vi "Global Variables.vi"() -> ()   [LabVIEW 2018]
panel:
  out "TabletProtocol":string
  out "FanProtocol":string
  out "ResistanceProtocol":string
  out "GradeProtocol":string
  out "DistanceDriver":string
  out "SpeedProtocol":string
  out "EnabledUSB":string
  in  "xmlParser 3":string[](array[string])=["Enabled", "SpeedProtocol", "DistanceDriver", "GradeProtocol", "ResistanceDriver", "FanProtocol", "TabletProtocol"]
  out "TVTest":string
  out "USBTest":string
  out "SoftwareVersion":string
  out "InclineCalibration":string
  out "Cosmetic":string
  out "Warning":string
  out "Finish":string
  out "CSAFETest":string
  out "AudioTest":string
  out "FanTest":string
  out "PulseTest":string
  out "ResistanceTest":string
  out "InclineTest":string
  out "TachInputTest":string
  out "PWMTest":string
  out "ButtonTest":string
  out "DisplayTest":string
  out "SafetyKey":string
  out "PowerUp":string
  out "Setup":string
  out "EquipmentNeeded":string
  out "BLETest":string
  out "BLESetup":string
  out "Firmware":string
  out "DisplayType":string
  out "CurrentLimit":string
  out "ConsoleVoltage":string
  out "Controller":string
  out "Description":string
  out "Units":string
  out "ProductType":string
  out "MCU":string
  out "PartNumber":string
  out "xPulse":i32
  out "yTV":i32
  out "xTV":i32
  out "yAudio":i32
  out "xAudio":i32
  out "y2Pulse":i32
  out "y1Pulse":i32
  out "advanceButton":i32
  out "modeButton":i32
  out "xmlFeature2":string[][](array[string])
  out "xmlData":string[](array[string])
  out "xmlFeature1":string[](array[string])
  in  "xmlParser 2":string[](array[string])=["MaxSpeed", "MinGrade", "MaxGrade", "TransMax", "DistanceDriver", "FanProtocol", "TabletProtocol"]
  in  "xmlParser 1":string[](array[string])=["consolePartNumber", "mcuChipName", "equipmentType", "systemUnitType", "BuildModelString", "PowerBoard", "ConsoleVoltage", "MaxCurrent"]
  in  "xmlParser 0":string[](array[string])=["SystemInfo/", "Display/TypeName", "ReleaseArray/ReleaseItem/GithubLink", "FeatureArray/FeatureItem", "FeatureArray/FeatureItem/", "KeyArray/KeyObj/MembraneKeyCode/KeyCodeValue", "AudioSources/AudioSrcItem", "PulseDriverArray/PulseDriverItem"]
  in  "jsonGen":string[](array[string])=["PartNumber", "Description", "ProductType", "DisplayType", "EquipmentNeeded", "Setup", "BLESetup", "Cosmetic", "PowerUp", "SafetyKey", "BLETest", "SoftwareVersion", "InclineCalibration", "DisplayTest", "ButtonTest", "PWMTest", "TachInputTest", "InclineTest", "ResistanceTest", "USBTest", "PulseTest", "FanTest", "AudioTest", "TVTest", "CSAFETest", "Finish"]
  # "Not used. Save this for other functions"
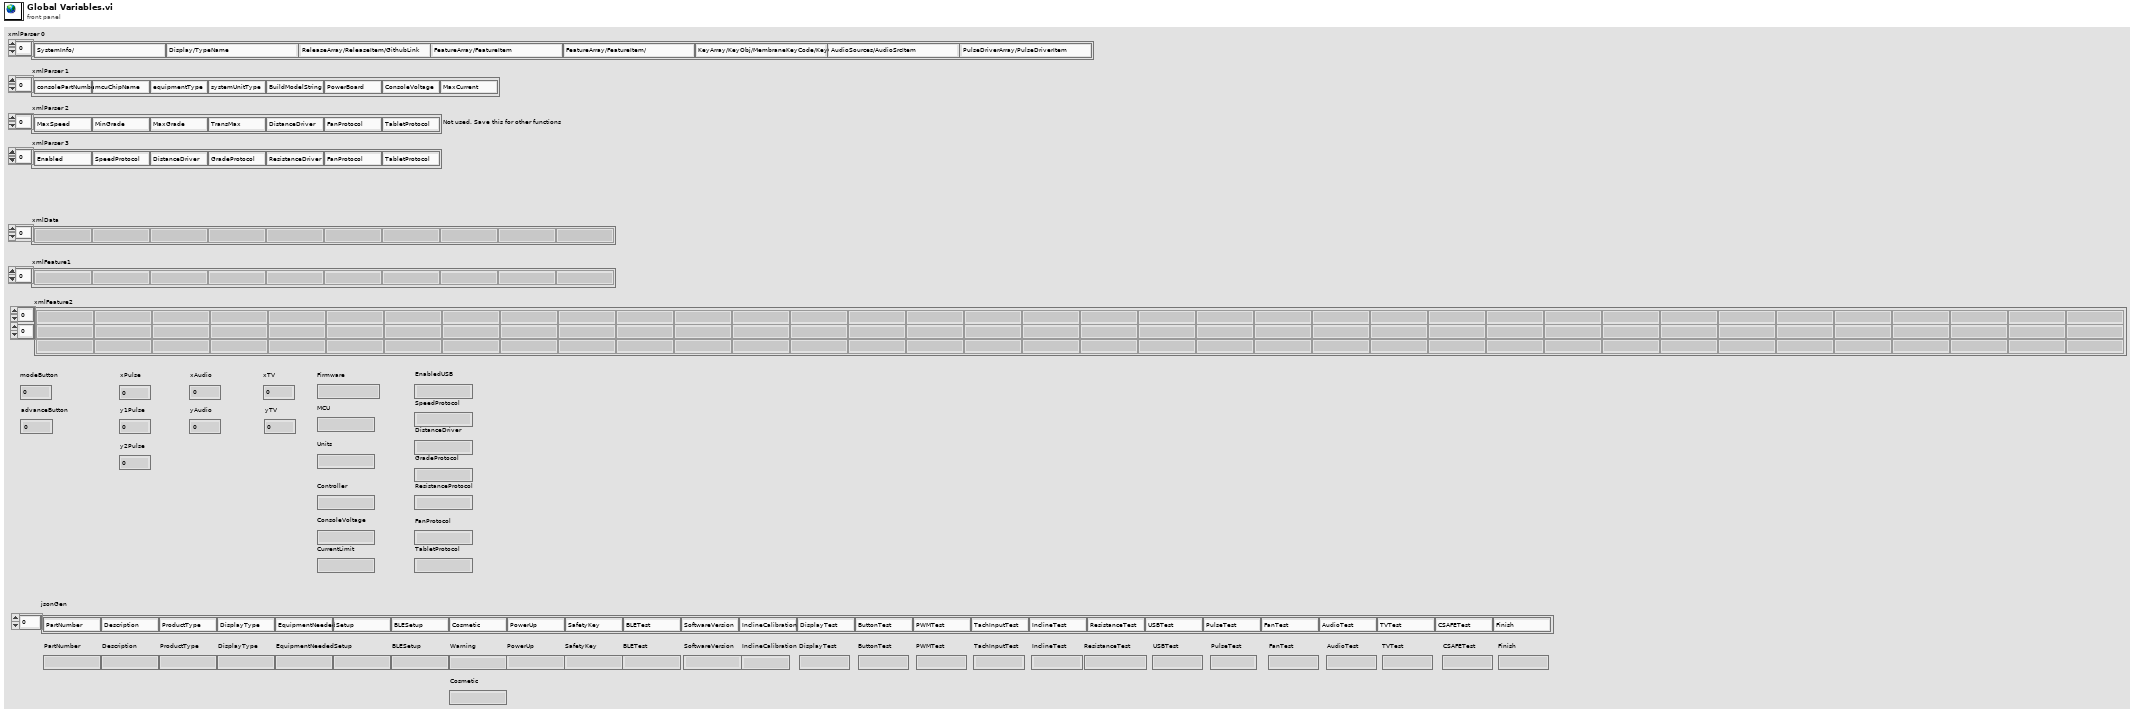
[diagram p1: front panel]
diagram:
